vi "Robot Main.vi"() -> ()   [LabVIEW 2016]
doc: "This VI implements the framework and scheduler for your robotics program. It should not be necessary to modify the framework. You are expected to add your code to the VIs called from Robot Main - the ones located in the Team Code folder within the project."
uses:
  Constants/Constants.lvlib
  SubSystems/Drive/Drive System.lvlib
  Constants/Private/Private Global.vi
  Vision/Vision Server/Vision Server.lvclass
  SubSystems/Path Track/Path Track.lvlib
  SubSystems/Intake/Intake.lvlib
  Vision/Vision Drive/Vision Drive.lvlib
panel:
  in  "Finish":bool
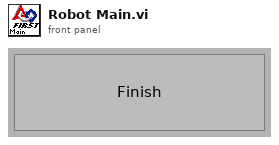
[diagram p1: front panel]
types:
  T1 = typedef "WPI_DriverStationMatch Info.ctl" = cluster{"Autonomous Elapsed Seconds":dbl, "TeleOp Elapsed Seconds":dbl, "Disabled Elapsed Seconds":dbl, "Visited Autonomous":bool, "Visited TeleOp":bool, "Visited Disabled":bool, "Autonomous Settings":cluster{"Autonomous Style":enum16{"Iterative", "Independent"}, "VI Refnum":refnum<vi>}}
  T2 = typedef "WPI_DriverStationDerivedRobotMode.ctl" = enum16{"Init", "Execute", "Stop"}
  T3 = typedef "WPI_DriverStationRobotMode2.ctl" = enum16{"Autonomous Disabled", "Autonomous Enabled", "Teleop Disabled", "Teleop Enabled", "Disconnected", "Finish", "Test Disabled", "Test Enabled", "Emergency Stopped"}
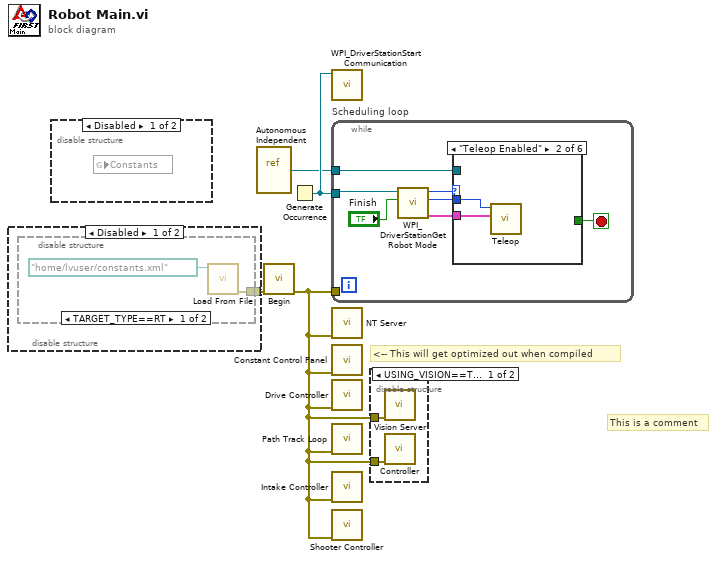
[diagram p0: block diagram]
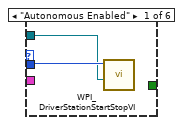
[diagram p5: hidden frame]
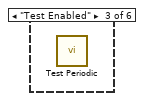
[diagram p6: hidden frame]
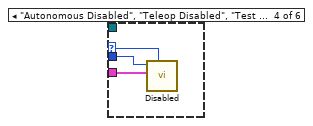
[diagram p7: hidden frame]
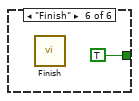
[diagram p9: hidden frame]
diagram:
  # "This is a comment"
  # "<-- This will get optimized out when compiled"
  n1 = disable-structure shown="Disabled" {
    disable-tunnel: [w5 _] -> w3
    frame Disabled {
      n2 = disable-structure shown="TARGET_TYPE==RT" {
        disable-tunnel: [w7 _] -> w5
        frame condition #0 (active) {
          n3 = call "Load From File.vi"("file"=path "/home/lvuser/constants.xml") -> ("error out"=w7:errorcluster)  [unwired: 10 in]
        }
        frame condition #1 {
        }
      }
    }
    frame Enabled {
    }
  }
  n4 = disable-structure shown="Disabled" {
    frame Disabled {
      n5 = global read "Private Global.vi" "Constants"() -> ()  [unwired: 1 in]
    }
    frame Enabled {
    }
  }
  n6 = vi-ref "Autonomous Independent.vi"() -> (w2:refnum<vi>)
  n7 = call "Begin.vi"("error in"=w3) -> ("error out"=w1:errorcluster)  [unwired: 1 in, 9 out]
  n8 = Generate Occurrence() -> (w4:refnum<k4>)
  n9 = call <vilib>:"WPI_DriverStationStart Communication.vi"("occurrence"=w4) -> ()  [unwired: 1 in, 10 out]
  n10 = while "Scheduling loop" {
    tunnel: w4 -> [w13]
    tunnel: w1 -> [_]
    tunnel: w2 -> [w8]
    stop <- w10 stop-if-true
    n11 = call <vilib>:"WPI_DriverStationGet Robot Mode.vi"("Finish"="Finish", "DS Occurrence"=w13) -> ("Match Info out"=w11:T1, "Call Context"=w14:T2, "Robot Mode"=w9:T3)  [unwired: 7 out]
    n12 = case shown="\"Teleop Enabled\"" w9 {
      selector: w9 -> [_ _ _ w19 _ _]
      tunnel: w14 -> [w16 w18 _ w21 _ _]
      tunnel: w11 -> [_ w17 _ w20 _ _]
      tunnel: [_ _ _ _ _ TRUE] -> w10
      tunnel: w8 -> [w15 _ _ _ _ _]
      frame "Autonomous Enabled" {
        n13 = call <vilib>:"WPI_DriverStationStartStopVI.vi"("VI in"=w15, "Call Context"=w16) -> ()  [unwired: 10 in]
      }
      frame "Teleop Enabled" {
        n14 = call "Teleop.vi"("Match Info"=w17, "Call Context"=w18) -> ()  [unwired: 1 in, 9 out]
      }
      frame "Test Enabled" {
        n15 = call "Test Periodic.vi"() -> ()  [unwired: 12 in]
      }
      frame "Autonomous Disabled", "Teleop Disabled", "Test Disabled" {
        n16 = call "Disabled.vi"("Robot Mode"=w19, "Match Info"=w20, "Call Context"=w21) -> ()  [unwired: 1 in, 8 out]
      }
      frame "Disconnected", Default {
      }
      frame "Finish" {
        n17 = call "Finish.vi"() -> ()  [unwired: 1 in, 7 out]
      }
    }
  }
  n18 = call <vilib>:"NT Server.vi"("error in (no error)"=w1) -> ()  [unwired: 11 in]
  n19 = call "Constant Control Panel.vi"("error in (no error)"=w1) -> ()  [unwired: 11 in]
  n20 = call "Drive Controller.vi"("error out"=w1) -> ()  [unwired: 11 in]
  n21 = call "Path Track Loop.vi"("error in"=w1) -> ()  [unwired: 11 in]
  n22 = call "Intake Controller.vi"("error in"=w1) -> ()  [unwired: 11 in]
  n23 = call "Shooter Controller.vi"("error in (no error)"=w1) -> ()  [unwired: 11 in]
  n24 = disable-structure shown="USING_VISION==TRUE" {
    disable-tunnel: w1 -> [w24 _]
    disable-tunnel: w1 -> [w23 _]
    frame condition #0 (active) {
      n25 = call "Vision Server.vi"("error in"=w24) -> ()  [unwired: 10 in, 1 out]
      n26 = call "Controller.vi"("error in"=w23) -> ()  [unwired: 11 in]
    }
    frame condition #1 {
    }
  }
